vi "PC Streaming Host with slow.vi"() -> ()   [LabVIEW 2012]
uses:
  <vilib>/userdefined/High Color/nirio_resource_hc.ctl
  hv cluster control.ctl
  <vilib>/FPGAPlugInAG/PXI-7951R/niLvFpga_Open_PXI-7951R.vi
  <vilib>/rvi/interface/common/dynamic/niFpgaDynamicAddResources.vi
  <vilib>/Utility/error.llb/Error Cluster From Error Code.vi
  <vilib>/rvi/errors/niLvFpgaAdjustHostInterfaceError.vi
  <vilib>/FPGAPlugInAG/Dynamic/niLvFpga_Close_Dynamic.vi
  <vilib>/rvi/interface/nirviOpenFPGA/nirviOpenFPGA.xnode
  FPGA Bitfiles/TopLevelFPGA3.0.lvbitx
  <vilib>/rvi/interface/nirviReadWriteControl/nirviReadWriteControl.xnode
  <vilib>/rvi/interface/nirviMethod/nirviMethod.xnode
  <vilib>/rvi/interface/nirviCloseFPGA/nirviCloseFPGA.xnode
  <vilib>/ptbypt/NI_PtbyPt.lvlib
  <vilib>/rvi/interface/Simulation/niFpgaSimulationCallBeginRW.vi
  RT_binary.vi
  NiFpgaLv.dll
  <vilib>/FPGAPlugInAG/Dynamic/niLvFpga_ReadFifo_Dynamic.vi
  <vilib>/rvi/errors/niLvFpgaMergeErrorWithErrorCode.vi
  CAENHVs/CAEN/labview/CAENHVWrapper/CAENHVWrapper.lvlib
panel:
  in  "Channel Cluster":T1={"det_type"=["", "", "", "", "", "", "", ""], "Serial numbers"=["", "", "", "", "", "", "", ""], "Sources"=["", "", "", "", "", "", "", ""], "Trigger level"=[4000, 4000, 4000, 4000, 4000, 4000, 4000, 4000], "Data Record On/Off"=[FALSE, FALSE, FALSE, FALSE, FALSE, FALSE, FALSE, FALSE, TRUE, FALSE, FALSE, FALSE, FALSE, FALSE, FALSE, TRUE], "Number of Channels"=8}
  in  "HV Cluster":T2={"HV Power On/Off"=[TRUE, TRUE], "Set Voltage"=["0", "0", "0", "0", "0", "0", "0", "0"], "HV Tolerance (%)"=1.0}
  out "created path":path
  out "File name":string
  out "Total Data Chunks to Write":dbl
  in  "Tab Control":T3(tab)
  in  "Write mode":bool
  out "directory exists - please wait":u8(slide)
  out "directory ok":bool
  in  "Write Enable":bool
  in  "File Path":path=path "D:/Users/reuterc/Desktop"
  out "File Writing Progress (%)":dbl(slide) scale=0.0..100.0
  in  "Slow Control On":bool
  in  "Fast Data On":bool
  in  "Number of Files to Write":u32=1
  in  "IP Address of NIST Time Server":string(combo)
  in  "VISA resource name":refnum<visa-resource-name>="COM3"
  in  "HV Power On/Off":bool[](array[boolean])=[FALSE, FALSE, FALSE, FALSE, FALSE, FALSE, FALSE, FALSE]
  in  "HV Tolerance (%)":dbl=1.0
  out "HV":sgl[](array[numeric])
  in  "IP adress HV2":string="1_0_0"
  in  "IP adress HV1":string="0_0_0"
  out "error HV":errorcluster
  in  "Set Voltage":string[](array[string])=["0", "0", "0", "0", "0", "0", "0", "0"]
  out "handle HV1":i32
  out "handle HV2":i32
  in  "General Cluster":cluster{"Location":i16} {"Location" items=["Purdue", "NIKHEF", "Zurich", "???"]}
  in  "PXI address":T4 caption="RIO Device"
  in  "det_type":string[](array[combo])=["", "", "", "", "", "", "", ""]
  in  "Serial numbers":string[](array[combo])=["", "", "", "", "", "", "", ""]
  in  "Sources":string[](array[combo])=["", "", "", "", "", "", "", ""]
  in  "Trigger level":i16[](array[numeric])=[4000, 4000, 4000, 4000, 4000, 4000, 4000, 4000] caption="Trigger"
  in  "Data Record On/Off":bool[](array[boolean])=[FALSE, FALSE, FALSE, FALSE, FALSE, FALSE, FALSE, FALSE]
  in  "Testpulse Cluster":T5={"Master Pulser On/Off"=FALSE, "Testpulse Turnaround Time (samples)"=14, "Pulse Separation (samples)"=0, "Pulse duration (samples)"=0}
  out "Samples per Data Chunk":u32
  in  "DAQ Info Cluster":T6={"Data Chunks per File"=1000, "Samples per Waveform"=95, "Pretrigger Samples"=15, "circular buffer length (samples)"=1000, "Waveforms per Data Chunk"=5000} {"Waveforms per Data Chunk" format="%.2p"}
  out "Average Throughput":dbl(graph)
  out "Loop Time":u32
  out "Inst. Throughput":dbl format="%#_6p"
  out "Elements in FIFO":u32(graph)
  out "FIFO Overflow":bool
  out "Current Chunk":u32
  out "Current File":i32
  out "Waveform Graph":dynamicdata(graph)
  out "Channel number displayed":i16=-1
  in  "Arduino read rate (Hz)":dbl=1.0
  out "Slow time":u64
  out "data":dbl[](array[numeric])
  in  "XON Character":u8=17 format="%.0x"
  in  "XOFF Character":u8=19 format="%.0x"
  out "Slow Cluster":T7
  out "read buffer":string
  out "Bad sensor?":string
  in  "Max Slow Entries per File":i32=86400
  out "Current Slow File":i32
  out "Current Slow Entry":i32
  out "Sensor out of bounds":bool
  out "Temperature":dbl(graph)
  out "Pressure":dbl(graph)
  out "magnetic field y coordinate":dbl(graph)
  out "total magnetic field":dbl(graph)
  out "magnetic field z coordinate":dbl(graph)
  out "magnetic field x coordinate":dbl(graph)
  out "humidity":dbl(graph)
  out "XML String":string
  out "Slow XML":string
  out "error out":errorcluster
  out "NIST Time":u64
  out "NIST Time Failed to Read":bool
  in  "Minutes to wait":u32=5 min=3
  out "UTC format":bool=TRUE
  out "FPGA Timestamp":u64
  out "Stopped":bool
  in  "stop 2":bool
  in  "stop":bool
  # "Channel 0"
  # "Channel 1"
  # "Channel 2"
  # "Channel 3"
  # "Channel 4"
  # "Channel 5"
  # "Channel 6"
  # "Channel 7"
  # "Write continuously"
  # "Write finite number of files"
  # "Program will stop when number of Files to Write is Complete OR if stop is pressed."
  # "TODO: Make this look like the \"detectors\" tab"
  # "Waveform/Data Chunk information"
  # "To compare directly on a scope: Horizontal scale: 200 ns/div Vertical scale: ~100 mV/div If 15 pretriggers, delay = 700 ns"
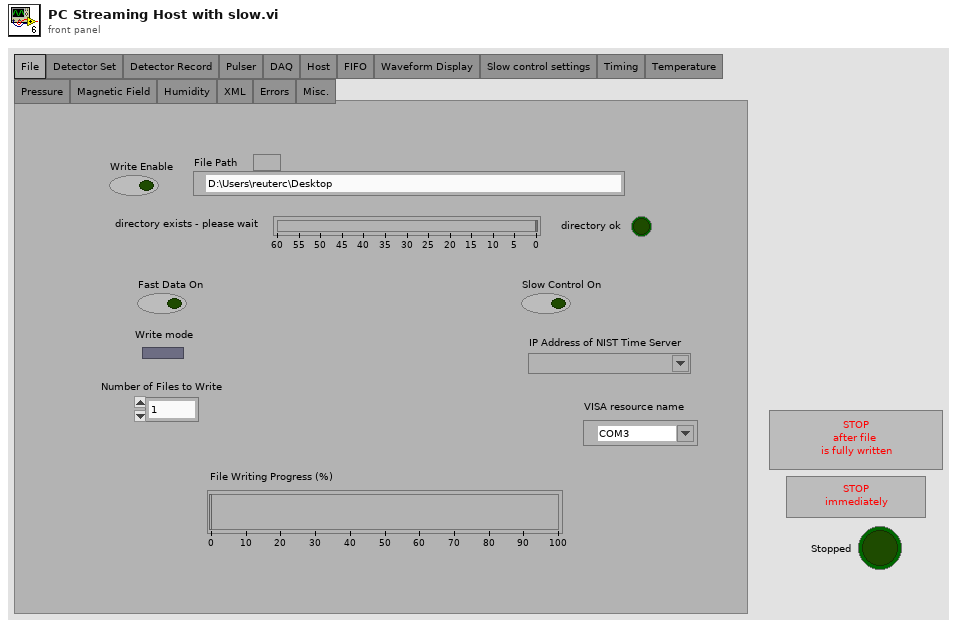
[diagram p1: front panel]
types:
  T1 = cluster{"det_type":string[], "Serial numbers":string[], "Sources":string[], "Trigger level":i16[], "Data Record On/Off":bool[], "Number of Channels":u8}
  T2 = typedef "hv cluster control.ctl" = cluster{"HV Power On/Off":bool[], "Set Voltage":string[], "HV Tolerance (%)":dbl}
  T3 = enum32{"File", "Detector Set", "Detector Record", "Pulser", "DAQ", "Host", "FIFO", "Waveform Display", "Slow control settings", "Timing", "Temperature", "Pressure", "Magnetic Field", "Humidity", "XML", "Errors", "Misc."}
  T4 = typedef "nirio_resource_hc.ctl" = tag
  T5 = cluster{"Master Pulser On/Off":bool, "Testpulse Turnaround Time (samples)":u32, "Pulse Separation (samples)":u32, "Pulse duration (samples)":u32}
  T6 = cluster{"Data Chunks per File":u32, "Samples per Waveform":u32, "Pretrigger Samples":u32, "circular buffer length (samples)":u32, "Waveforms per Data Chunk":u32}
  T7 = cluster{"Arduino Parameters":dbl, "Total Number of Slow Parameters":i32, "UTC format?":bool, "Sensor Upper bounds":i32[], "Sensor Lower bounds":i32[], "Descriptions":string[], "datanames":string[]}
  T8 = enum16{"open", "replace", "create", "open or create", "replace or create", "replace or create with confirmation"}
  T9 = enum16{"big-endian, network order", "native, host order", "little-endian"}
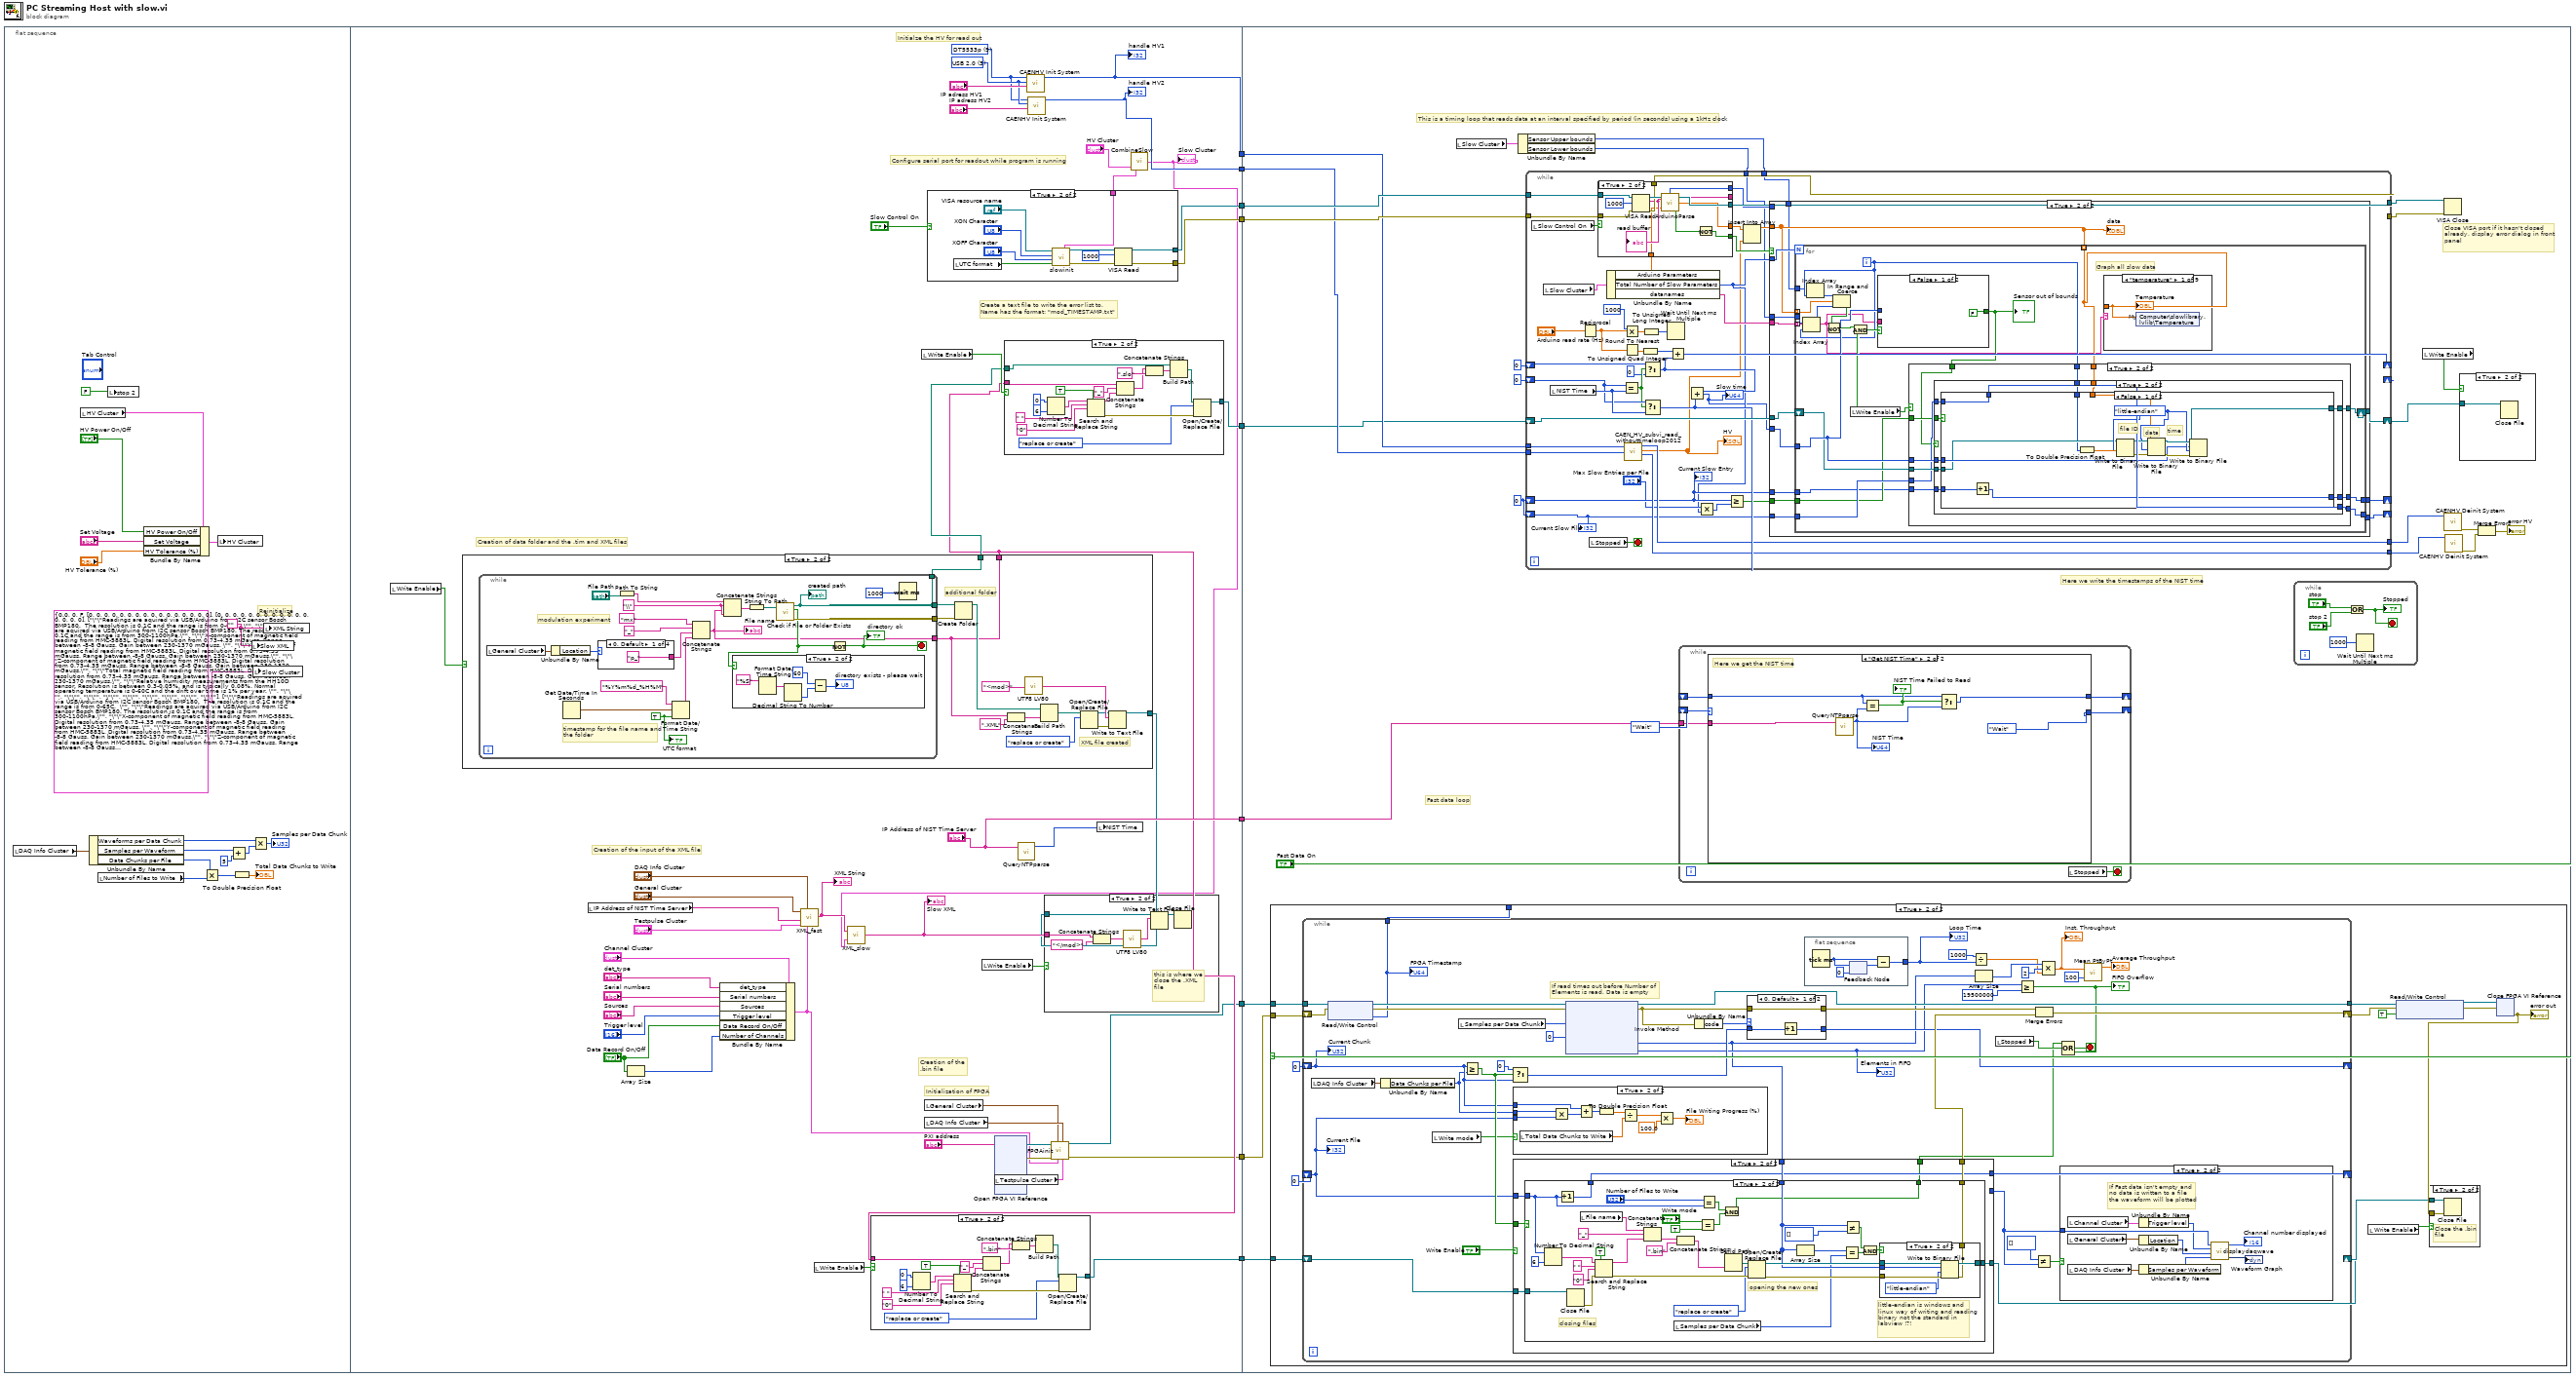
[diagram p0: block diagram]
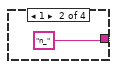
[diagram p7: hidden frame]
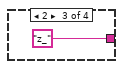
[diagram p8: hidden frame]
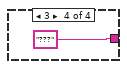
[diagram p9: hidden frame]
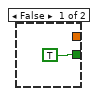
[diagram p11: hidden frame]
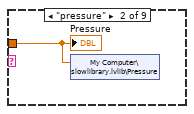
[diagram p13: hidden frame]
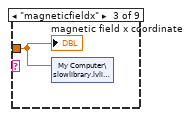
[diagram p14: hidden frame]
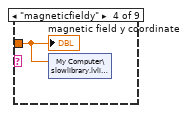
[diagram p15: hidden frame]
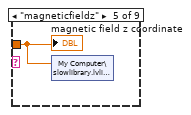
[diagram p16: hidden frame]
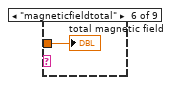
[diagram p17: hidden frame]
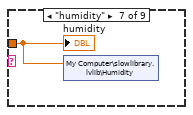
[diagram p18: hidden frame]
diagram:
  n1 = flat-sequence {
    tunnel: ["IP Address of NIST Time Server"] -> w9
    tunnel: [w48] -> w8
    tunnel: [w47] -> w7
    tunnel: [w43] -> w6
    tunnel: [w42] -> w5
    tunnel: [w41] -> w4
    tunnel: [w32] -> w3
    tunnel: [w31] -> w2
    tunnel: [w30] -> w1
    tunnel: w9 -> [w183]
    tunnel: w8 -> [w172]
    tunnel: w7 -> [w171]
    tunnel: w6 -> [w168]
    tunnel: w5 -> [w170]
    tunnel: w4 -> [w169]
    tunnel: w3 -> [w167]
    tunnel: w2 -> [w166]
    tunnel: w1 -> [w165]
    frame #0 {
      w26 = ""
      # "Reinitialize"
      n2 = local read "DAQ Info Cluster"() -> (w19:T6)
      n3 = local read "HV Cluster"() -> (w22:T2)
      n4 = Unbundle By Name(w19) -> ("Waveforms per Data Chunk"=w11:u32, "Samples per Waveform"=w12:u32, "Data Chunks per File"=w13:u32)
      n5 = local read "Number of Files to Write"() -> (w14:u32)
      n6 = local write "stop 2"(FALSE ("stop 2")) -> ()
      n7 = Bundle By Name(cluster=w22, "HV Power On/Off"="HV Power On/Off", "Set Voltage"="Set Voltage", "HV Tolerance (%)"="HV Tolerance (%)") -> (w24:T2)
      n8 = Multiply(x=w13, y=w14) -> (x*y=w18:u32)
      n9 = local write "HV Cluster"(w24) -> ()
      n10 = Add(x=w12, y=u32 5) -> (x+y=w16:u32)
      n11 = To Double Precision Float(number=w18) -> (double precision float=→"Total Data Chunks to Write":dbl)
      n12 = local write "Slow XML"(w26) -> ()
      n13 = Multiply(x=w11, y=w16) -> (x*y=→"Samples per Data Chunk":u32)
      n14 = local write "Slow Cluster"(T7 {"Arduino Parameters"=0.0, "Total Number of Slow Parameters"=0, "UTC format?"=FALSE, "Sensor Upper bounds"=[0, 0, 0, 0, 0, 0, 0, 0, 0, 0, 0, 0, 0, 0, 0, 0], "Sensor Lower bounds"=[0, 0, 0, 0, 0, 0, 0, 0, 0, 0, 0, 0, 0, 0, 0, 0], "Descriptions"=["\"\"Readings are aquired via USB/Arduino from I2C sensor Bosch BMP180.  The resolution is 0.1C and the range is from 0-65C.  \"", "\"\"Readings are aquired via USB/Arduino from I2C sensor Bosch BMP180. The resolution is 0.1C and the range is from 300-1100hPa.\"", "\"\"X-component of magnetic field reading from HMC-5883L. Digital resolution from 0.73-4.35 mGauss. Range between -8-8 Gauss. Gain between 230-1370 mGauss. \"", "\"\"Y-component of magnetic field reading from HMC-5883L. Digital resolution from 0.73-4.35 mGauss. Range between -8-8 Gauss. Gain between 230-1370 mGauss.\"", "\"\"Z-component of magnetic field reading from HMC-5883L. Digital resolution from 0.73-4.35 mGauss. Range between -8-8 Gauss. Gain between 230-1370 mGauss.\"", "\"\"Total magnetic field reading from HMC-5883L. Digital resolution from 0.73-4.35 mGauss. Range between -8-8 Gauss. Gain between 230-1370 mGauss.\"", "\"\"Relative humidity measurements from the HH10D sensor. Resolution is between 0.3-0.05%, and is typically 0.08%. Normal operating temperature is 0-60C and the drift over time is 1% per year. \"", "\"\"", "\"\"", "\"\"", "\"\"", "\"\"", "\"\"", "\"\"", "\"\"", "\"\""], "datanames"=["\"\"Readings are aquired via USB/Arduino from I2C sensor Bosch BMP180.  The resolution is 0.1C and the range is from 0-65C.  \"", "\"\"Readings are aquired via USB/Arduino from I2C sensor Bosch BMP180. The resolution is 0.1C and the range is from 300-1100hPa.\"", "\"\"X-component of magnetic field reading from HMC-5883L. Digital resolution from 0.73-4.35 mGauss. Range between -8-8 Gauss. Gain between 230-1370 mGauss. \"", "\"\"Y-component of magnetic field reading from HMC-5883L. Digital resolution from 0.73-4.35 mGauss. Range between -8-8 Gauss. Gain between 230-1370 mGauss.\"", "\"\"Z-component of magnetic field reading from HMC-5883L. Digital resolution from 0.73-4.35 mGauss. Range between -8-8 Gauss. Gain between 230-1370 mGauss.\"", "\"\"Total magnetic field reading from HMC-5883L. Digital resolution from 0.73-4.35 mGauss. Range between -8-8 Gauss. Gain between 230-1370 mGauss.\"", "\"\"Relative humidity measurements from the HH10D sensor. Resolution is between 0.3-0.05%, and is typically 0.08%. Normal operating temperature is 0-60C and the drift over time is 1% per year. \"", "\"\"", "\"\"", "\"\"", "\"\"", "\"\"", "\"\"", "\"\"", "\"\"", "\"\""]} ("Cluster")) -> ()
      n15 = local write "XML String"(w26) -> ()
    }
    frame #1 {
      w50 = 3 items=["TCP/IP"=0, "HS CAENET"=2, "USB 2.0"=3, "CONET Optical Link"=4, "USB VCP"=5] ("LinkType")
      w49 = u32 9 items=["SY1527", "SY2527", "SY4527", "SY5527", "N568", "V65XX", "N1470", "V8100", "", "DT5533p"] ("system")
      # "Initialization of FPGA"
      # "Creation of the \n.bin file"
      # "Initialze the HV for read out"
      # "Create a text file to write the error list to.  \nName has the format: \"mod_TIMESTAMP.txt\""
      # "Creation of the input of the XML file"
      # "Configure serial port for readout while program is running"
      # "Creation of data folder and the .tim and XML files"
      n16 = local read "Write Enable"() -> (w72:bool)
      n17 = case shown="True" w72 {
        tunnel: [_ w133] -> w44
        tunnel: [_ w125] -> w46
        tunnel: [_ w122] -> w33
        frame False {
        }
        frame True {
          # "XML file created"
          # "additional folder"
          n18 = while {
            tunnel: [w148] -> w134
            tunnel: [w140] -> w135
            tunnel: [w140] -> w133
            tunnel: [w139] -> w122
            stop <- w145 stop-if-true
            w141 = "\\" ("string")
            w151 = TRUE ("UTC format")
            # "modulation experiment"
            # "timestamp for the file name and the folder"
            n19 = local read "General Cluster"() -> (w137:cluster{"Location":i16})
            n20 = Unbundle By Name(w137) -> ("Location"=w136:i16)
            n21 = Get Date/Time In Seconds() -> (seconds since 1Jan1904=w152:timestamp)
            n22 = case shown="0, Default" w136 {
              tunnel: ["p_" ("string") "n_" ("string") "z_" ("string") "???"] -> w138
              frame 0, Default {
              }
              frame 1 {
              }
              frame 2 {
              }
              frame 3 {
              }
            }
            n23 = Path To String(path="File Path") -> (string=w154:string)
            n24 = Format Date/Time String(time format string (%c)="%Y%m%d_%H%M", seconds (now)=w152, UTC format=w151) -> (date/time string=w142:string)
            n25 = Concatenate Strings("mx" ("string"), "_" ("string"), w138, w142) -> (w139:string)
            "File name" <- w139
            n26 = Concatenate Strings(w154, w141, w139, w141) -> (w155:string)
            n27 = String To Path(string=w155) -> (path=w149:path)
            n28 = call <vilib>:"Check if File or Folder Exists.vi"("path"=w149) -> ("error out"=w148:errorcluster, "file or folder exists?"=w147:bool, "dup path"=w140:path)  [unwired: 8 in]
            "created path" <- w140
            n29 = case shown="True" w147 {
              frame False {
              }
              frame True {
                n30 = Format Date/Time String(time format string (%c)="%S") -> (date/time string=w163:string)  [unwired: 2 in]
                n31 = Decimal String To Number(string=w163) -> (number=w161:i32)  [unwired: 2 in, 1 out]
                n32 = Subtract(x=60, y=w161) -> (x-y=→"directory exists - please wait":i32)
              }
            }
            n33 = Not(x=w147) -> (.not. x?=w145:bool)
            "directory ok" <- w145
            n34 = Wait (ms)(milliseconds to wait=1000) -> ()  [unwired: 1 out]
            "UTC format" <- w151
          }
          n35 = Create Folder(path (use dialog)=w135, error in=w134) -> (created path=w123:path)  [unwired: 1 in, 2 out]
          n36 = Concatenate Strings(w122, ".XML" ("substring (\"\")")) -> (w129:string)
          n37 = call "UTF8 LV80.vi"("text"="<mod>") -> ("utf-8 text out"=w132:string)
          n38 = Build Path(base path=w123, name or relative path=w129) -> (appended path=w128:path)
          n39 = Open/Create/Replace File(file path (use dialog)=w128, operation (0:open)=T8."replace or create") -> (refnum out=w131:refnum<file>, error out=w130:errorcluster)  [unwired: 4 in, 1 out]
          n40 = Write to Text File(file (use dialog)=w131, text=w132, error in=w130) -> (refnum out=w125:refnum<file>)  [unwired: 1 in, 2 out]
        }
      }
      n41 = local read "IP Address of NIST Time Server"() -> (w62:string)
      n42 = Array Size(array="Data Record On/Off") -> (size(s)=w60:i32)
      n43 = Bundle By Name(cluster="Channel Cluster", "det_type"="det_type", "Serial numbers"="Serial numbers", "Sources"="Sources", "Trigger level"="Trigger level", "Data Record On/Off"="Data Record On/Off", "Number of Channels"=w60) -> (w29:T1)
      n44 = call "XML_fast.vi"("Channel Cluster"=w29, "DAQ Info Cluster"="DAQ Info Cluster", "Testpulse Cluster"="Testpulse Cluster", "IP Address of NIST Time Server"=w62, "General Cluster"="General Cluster") -> ("XML String"=w65:string)  [unwired: 6 in]
      "XML String" <- w65
      n45 = local read "Write Enable"() -> (w34:bool)
      n46 = case shown="True" w34 {
        tunnel: [_ w81] -> w32
        tunnel: w33 -> [_ w73]
        frame False {
        }
        frame True {
          n47 = Number To Decimal String(number=0, width (-)=i16 6) -> (decimal integer string=w88:string)
          n48 = Search and Replace String(replace all?=TRUE ("replace all? (F)"), input string=w88, search string=" ", replace string="0" ("replace string (\"\")")) -> (result string=w78:string, error out=w83:errorcluster)  [unwired: 4 in, 2 out]
          n49 = Concatenate Strings(w73, "_" ("string"), w78) -> (w76:string)
          n50 = Concatenate Strings(w76, ".bin" ("substring (\"\")")) -> (w80:string)
          n51 = Build Path(name or relative path=w80) -> (appended path=w84:path)  [unwired: 1 in]
          n52 = Open/Create/Replace File(file path (use dialog)=w84, error in=w83, operation (0:open)=T8."replace or create") -> (refnum out=w81:refnum<file>)  [unwired: 3 in, 2 out]
        }
      }
      n53 = local read "Write Enable"() -> (w45:bool)
      n54 = local read "General Cluster"() -> (w37:cluster{"Location":i16})
      n55 = local read "DAQ Info Cluster"() -> (w38:T6)
      n56 = case shown="True" "Slow Control On" {
        tunnel: [_ w121] -> w48
        tunnel: [_ w120] -> w47
        tunnel: [_ w112] -> w71
        frame False {
        }
        frame True {
          n57 = local read "UTC format"() -> (w115:bool)
          n58 = call "slowinit.vi"("UTC format"=w115, "XOFF Character"="XOFF Character", "XON Character"="XON Character", "VISA resource name"="VISA resource name") -> ("error IO"=w113:errorcluster, "VISA resource name out"=w114:refnum<visa-resource-name>, "Slow Cluster"=w112:T7)  [unwired: 5 in]
          n59 = VISA Read(VISA resource name=w114, byte count=u32 1000, error in (no error)=w113) -> (VISA resource name out=w121:refnum<visa-resource-name>, error out=w120:errorcluster)  [unwired: 2 out]
        }
      }
      n60 = local read "Write Enable"() -> (w53:bool)
      n61 = local read "Testpulse Cluster"() -> (w36:T5)
      n62 = xnode "Open FPGA VI Reference"("resource name"="PXI address") -> ("FPGA VI Reference Out"=w40:refnum<k20>, "error out"=w39:errorcluster)  [unwired: 1 in]
      n63 = case shown="True" w45 {
        tunnel: [_ w98] -> w43
        tunnel: w33 -> [_ w90]
        tunnel: w44 -> [_ w89]
        frame False {
        }
        frame True {
          n64 = Number To Decimal String(number=0, width (-)=i16 6) -> (decimal integer string=w105:string)
          n65 = Search and Replace String(replace all?=TRUE ("replace all? (F)"), input string=w105, search string=" ", replace string="0" ("replace string (\"\")")) -> (result string=w95:string, error out=w100:errorcluster)  [unwired: 4 in, 2 out]
          n66 = Concatenate Strings(w90, "_" ("string"), w95) -> (w93:string)
          n67 = Concatenate Strings(w93, ".slo" ("substring (\"\")")) -> (w97:string)
          n68 = Build Path(base path=w89, name or relative path=w97) -> (appended path=w101:path)
          n69 = Open/Create/Replace File(file path (use dialog)=w101, error in=w100, operation (0:open)=T8."replace or create") -> (refnum out=w98:refnum<file>)  [unwired: 3 in, 2 out]
        }
      }
      n70 = call "QueryNTPparse.vi"("IP Address of NIST Server"="IP Address of NIST Time Server") -> ("NTP Time"=w68:u64)  [unwired: 1 in, 2 out]
      n71 = call "CAENHV Init System.vi"("Arg"="IP adress HV1", "LinkType"=w50, "system"=w49) -> ("handle"=w42:i32)  [unwired: 7 in, 1 out]
      "handle HV1" <- w42
      n72 = call "CAENHV Init System.vi"("Arg"="IP adress HV2", "LinkType"=w50, "system"=w49) -> ("handle"=w41:i32)  [unwired: 7 in, 1 out]
      "handle HV2" <- w41
      n73 = call "FPGAinit.vi"("Testpulse Cluster"=w36, "DAQ Info Cluster"=w38, "Channel Cluster"=w29, "General Cluster"=w37, "error in"=w39, "FPGA VI Reference In"=w40) -> ("error out"=w30:errorcluster, "FPGA VI Reference Out"=w31:refnum<k20>)  [unwired: 4 in]
      n74 = local write "NIST Time"(w68) -> ()
      n75 = call "CombineSlow.vi"("HV Cluster"="HV Cluster", "Slow Cluster"=w71) -> ("Slow Cluster 2"=w28:T7)
      "Slow Cluster" <- w28
      n76 = call "XML_slow.vi"("Slow Cluster"=w28, "Input String"=w65) -> ("Output String"=w66:string)
      "Slow XML" <- w66
      n77 = case shown="True" w53 {
        tunnel: w46 -> [_ w111]
        tunnel: w66 -> [_ w106]
        frame False {
        }
        frame True {
          # "this is where we close the .XML file"
          n78 = Concatenate Strings(w106, "</mod>" ("string")) -> (w107:string)
          n79 = call "UTF8 LV80.vi"("text"=w107) -> ("utf-8 text out"=w110:string)
          n80 = Write to Text File(file (use dialog)=w111, text=w110) -> (refnum out=w109:refnum<file>)  [unwired: 2 in, 2 out]
          n81 = Close File(refnum=w109) -> ()  [unwired: 1 in, 2 out]
        }
      }
    }
    frame #2 {
      w173 = 0
      # "Fast data loop"
      # "This is a timing loop that reads data at an interval specified by period (in seconds) using a 1kHz clock"
      # "Close VISA port if it hasn't closed already, display error dialog in front panel"
      # "Here we write the timestamps of the NIST time"
      n82 = case shown="True" "Fast Data On" {
        tunnel: [_ w379] -> _
        tunnel: w167 -> [_ w375]
        tunnel: w166 -> [_ w374]
        tunnel: w165 -> [_ w373]
        frame False {
        }
        frame True {
          n83 = while {
            shift-right: [w416] -> w381
            shift-left: w373 -> [w405]
            shift-right: [w412] -> _
            shift-left: u32 0 -> [w409]
            shift-right: [w397] -> _
            shift-left: 0 ("number") -> [w398]
            shift-right: [w413] -> w383
            shift-left: w375 -> [w414]
            tunnel: [w432] -> w378
            tunnel: [w402] -> w379
            tunnel: w374 -> [w391]
            stop <- w399 stop-if-true
            # "If read times out before Number of Elements is read, Data is empty"
            n84 = local read "DAQ Info Cluster"() -> (w393:T6)
            n85 = xnode "Read/Write Control"("FPGA VI Reference In"=w391, "error in"=w405) -> ("FPGA VI Reference Out"=w404:refnum<k20>, "error out"=w403:errorcluster, "Timestamp"=w402:u64)
            "FPGA Timestamp" <- w402
            n86 = Unbundle By Name(w393) -> ("Data Chunks per File"=w392:u32)
            n87 = local read "Write mode"() -> (w406:bool)
            n88 = local read "Samples per Data Chunk"() -> (w390:u32)
            n89 = Greater Or Equal?(x=w409, y=w392) -> (x >= y?=w418:bool)
            n90 = Select(t=u32 0, s=w418, f=w409) -> (s? t:f=w419:u32)
            n91 = case shown="True" w406 {
              tunnel: w398 -> [_ w451]
              tunnel: w409 -> [_ w449]
              tunnel: w392 -> [_ w442]
              frame False {
              }
              frame True {
                n92 = local read "Total Data Chunks to Write"() -> (w446:dbl)
                n93 = Multiply(x=w442, y=w451) -> (x*y=w450:u32)
                n94 = Add(x=w449, y=w450) -> (x+y=w448:u32)
                n95 = To Double Precision Float(number=w448) -> (double precision float=w447:dbl)
                n96 = Divide(x=w447, y=w446) -> (x/y=w444:dbl)
                n97 = Multiply(x=w444, y=100.0) -> (x*y=→"File Writing Progress (%)":dbl)
              }
            }
            n98 = xnode "Invoke Method"("FPGA VI Reference In"=w404, "error in"=w403, "Number of Elements"=w390, "Timeout (ms)"=0) -> ("FPGA VI Reference Out"=w432:refnum<k20>, "error out"=w429:errorcluster, "Data"=w407:i16[], "Elements Remaining"=w408:u32)
            "Elements in FIFO" <- w408
            n99 = case shown="True" "Write Enable" {
              tunnel: w407 -> [w458 w463]
              tunnel: [w458 _] -> w396
              tunnel: w418 -> [_ w467]
              tunnel: [_ w466] -> w415
              tunnel: [w459 w465] -> w413
              tunnel: w414 -> [w459 w464]
              tunnel: w398 -> [w457 w462]
              tunnel: [w457 w461] -> w397
              tunnel: [FALSE w460] -> w389
              frame False {
              }
              frame True {
                n100 = case shown="True" w467 {
                  tunnel: w463 -> [w471 w495]
                  tunnel: [w470 w497] -> w466
                  tunnel: w464 -> [w475 w510]
                  tunnel: [w474 w503] -> w465
                  tunnel: w462 -> [w469 w484]
                  tunnel: [w469 w490] -> w461
                  tunnel: [FALSE w482] -> w460
                  frame False {
                    # "binary writing will write 0 if there is no data"
                    n101 = Not Equal?(x=w471, y=i16[] []) -> (x != y?=w472:bool)
                    n102 = case shown="True" w472 {
                      tunnel: w475 -> [w476 w481]
                      tunnel: [w476 w480] -> w474
                      tunnel: [_ w479] -> w470
                      tunnel: w471 -> [_ w477]
                      frame False {
                      }
                      frame True {
                        n103 = Write to Binary File(file (use dialog)=w481, data=w477, 9:T9."little-endian" ("byte order (0:big-endian, network order)")) -> (refnum out=w480:refnum<file>, error out=w479:errorcluster)  [unwired: 3 in, 1 out]
                      }
                    }
                  }
                  frame True {
                    # "little-endian is windows and linux way of writing and reading binary not the standard in labview !?!"
                    # "opening the new ones"
                    # "closing files"
                    n104 = Number To Decimal String(number=w484, width (-)=i16 6) -> (decimal integer string=w512:string)
                    n105 = Increment(x=w484) -> (x+1=w490:i32)
                    n106 = Close File(refnum=w510) -> (error out=w509:errorcluster)  [unwired: 1 in, 1 out]
                    n107 = local read "File name"() -> (w491:string)
                    n108 = Search and Replace String(replace all?=TRUE ("replace all? (F)"), input string=w512, search string=" ", replace string="0" ("replace string (\"\")"), error in=w509) -> (result string=w502:string, error out=w508:errorcluster)  [unwired: 3 in, 2 out]
                    n109 = Concatenate Strings(w491, "_" ("string"), w502) -> (w498:string)
                    n110 = local read "Samples per Data Chunk"() -> (w489:u32)
                    n111 = Concatenate Strings(w498, ".bin" ("substring (\"\")")) -> (w500:string)
                    n112 = Equal?(x="Write mode", y=TRUE) -> (x = y?=w488:bool)
                    n113 = Equal?(x="Number of Files to Write", y=w484) -> (x = y?=w487:bool)
                    n114 = And(x=w487, y=w488) -> (x .and. y?=w482:bool)
                    n115 = Build Path(name or relative path=w500) -> (appended path=w507:path)  [unwired: 1 in]
                    n116 = Open/Create/Replace File(file path (use dialog)=w507, error in=w508, operation (0:open)=T8."replace or create") -> (refnum out=w504:refnum<file>, error out=w505:errorcluster)  [unwired: 3 in, 1 out]
                    n117 = Array Size(array=w495) -> (size(s)=w494:i32)
                    n118 = Equal?(x=w494, y=w489) -> (x = y?=w493:bool)
                    n119 = Not Equal?(x=w495, y=i16[] []) -> (x != y?=w496:bool)
                    n120 = And(x=w496, y=w493) -> (x .and. y?=w492:bool)
                    n121 = case shown="True" w492 {
                      tunnel: w505 -> [w517 w524]
                      tunnel: w504 -> [w518 w523]
                      tunnel: [w518 w522] -> w503
                      tunnel: [w517 w521] -> w497
                      tunnel: w495 -> [_ w520]
                      frame False {
                      }
                      frame True {
                        n122 = Write to Binary File(file (use dialog)=w523, data=w520, error in=w524, 9:T9."little-endian" ("byte order (0:big-endian, network order)")) -> (refnum out=w522:refnum<file>, error out=w521:errorcluster)  [unwired: 2 in, 1 out]
                      }
                    }
                  }
                }
              }
            }
            n123 = Unbundle By Name(w429) -> ("code"=w430:i32)
            n124 = case shown="0, Default" w430 {
              tunnel: [w527 errorcluster {"status"=FALSE, "code"=0, "source"=""} ("error constant")] -> w417
              tunnel: w429 -> [w527 _]
              tunnel: w419 -> [w526 w528]
              tunnel: [w525 w528] -> w412
              frame 0, Default {
                n125 = Increment(x=w526) -> (x+1=w525:u32)
              }
              frame -50400 {
                # "Timeout"
              }
            }
            n126 = flat-sequence {
              tunnel: [w455] -> w423
              frame #0 {
                n127 = Tick Count (ms)() -> (millisecond timer value=w454:u32)
                n128 = feedback #1(u32 0 ("millisecond timer value")) -> (w453:u32)
                n129 = feedback-in #1(w454) -> ()
                n130 = Subtract(x=w454, y=w453) -> (x-y=w455:u32)
              }
            }
            n131 = Divide(x=u32 1000, y=w423) -> (x/y=w425:dbl)
            n132 = Array Size(array=w407) -> (size(s)=w428:i32)
            n133 = local read "Stopped"() -> (w401:bool)
            n134 = Greater Or Equal?(x=w408, y=u32 19500000) -> (x >= y?=w400:bool)
            "FIFO Overflow" <- w400
            n135 = Not Equal?(x=i16[] [], y=w396) -> (x != y?=w394:bool)
            n136 = Merge Errors(w417, w415) -> (w416:errorcluster)
            n137 = Compound Arithmetic op=MULTIPLY(w428, 2 ("y"), w425) -> (w422:dbl)
            "Inst. Throughput" <- w422
            n138 = case shown="True" w394 {
              tunnel: w396 -> [_ w441]
              frame False {
              }
              frame True {
                # "If Fast data isn't empty and\nno data is written to a file\nthe waveform will be plotted"
                n139 = local read "Channel Cluster"() -> (w439:T1)
                n140 = local read "General Cluster"() -> (w437:cluster{"Location":i16})
                n141 = local read "DAQ Info Cluster"() -> (w435:T6)
                n142 = Unbundle By Name(w439) -> ("Trigger level"=w438:i16[])
                n143 = Unbundle By Name(w437) -> ("Location"=w436:i16)
                n144 = Unbundle By Name(w435) -> ("Samples per Waveform"=w434:u32)
                n145 = call "displaydaqwave.vi"("Samples per Waveform"=w434, "Location"=w436, "Trigger level"=w438, "Waveform from DAQ"=w441) -> ("Waveform Graph"=→"Waveform Graph":dynamicdata, "Channel number displayed"=→"Channel number displayed":i16)  [unwired: 6 in]
              }
            }
            n146 = Compound Arithmetic op=OR(w389, w401, w400) -> (w399:bool)
            n147 = call <vilib>:"Mean PtByPt.vi"("x"=w422, "sample length"=100) -> ("mean"=→"Average Throughput":dbl)  [unwired: 2 in, 1 out]
            "Loop Time" <- w423
            "Current Chunk" <- w409
            "Current File" <- w398
          }
          n148 = local read "Write Enable"() -> (w385:bool)
          n149 = xnode "Read/Write Control"("FPGA VI Reference In"=w378, "error in"=w381, "Stop FPGA and exit"=TRUE) -> ("FPGA VI Reference Out"=w377:refnum<k20>, "error out"=w376:errorcluster)
          n150 = xnode "Close FPGA VI Reference"("FPGA VI Reference In"=w377, "error in"=w376) -> ("error out"=w386:errorcluster)
          "error out" <- w386
          n151 = case shown="True" w385 {
            tunnel: w386 -> [_ w387]
            tunnel: w383 -> [_ w388]
            frame False {
            }
            frame True {
              # "Close the .bin\nfile"
              n152 = Close File(refnum=w388, error in=w387) -> ()  [unwired: 2 out]
            }
          }
        }
      }
      n153 = local read "Slow Cluster"() -> (w187:T7)
      n154 = Unbundle By Name(w187) -> ("Sensor Upper bounds"=w177:i32[], "Sensor Lower bounds"=w176:i32[])
      n155 = while {
        tunnel: [w236] -> w179
        tunnel: [w235] -> w178
        shift-right: [w228] -> _
        shift-left: u64 0 ("NIST Time") -> [w232]
        shift-right: [w224] -> _
        shift-left: u64 0 -> [w230]
        tunnel: [w216] -> w181
        tunnel: [w215] -> w180
        shift-right: [w208] -> w182
        shift-left: w168 -> [w234]
        shift-right: [w204] -> _
        shift-left: w173 -> [w205]
        shift-right: [w203] -> _
        shift-left: w173 -> [w207]
        tunnel: w177 -> [w196]
        tunnel: w176 -> [w195]
        tunnel: w172 -> [w194]
        tunnel: w171 -> [w193]
        tunnel: w170 -> [w192]
        tunnel: w169 -> [w191]
        stop <- w227 stop-if-true
        n156 = local read "Slow Control On"() -> (w211:bool)
        n157 = local read "Slow Cluster"() -> (w218:T7)
        n158 = local read "NIST Time"() -> (w233:u64)
        n159 = Reciprocal(x="Arduino read rate (Hz)") -> (1/x=w221:dbl)
        n160 = local read "Stopped"() -> (w227:bool)
        n161 = Unbundle By Name(w218) -> ("Arduino Parameters"=w212:dbl, "Total Number of Slow Parameters"=w201:i32, "datanames"=w209:string[])
        n162 = case shown="True" w211 {
          tunnel: [_ w248] -> w236
          tunnel: [_ w247] -> w235
          tunnel: [_ w245] -> w217
          tunnel: [_ w244] -> _
          tunnel: [TRUE w240] -> w210
          tunnel: [_ w242] -> w214
          tunnel: w212 -> [_ w241]
          tunnel: w194 -> [_ w239]
          tunnel: w193 -> [_ w238]
          frame False {
          }
          frame True {
            n163 = VISA Read(VISA resource name=w239, byte count=u32 1000, error in (no error)=w238) -> (VISA resource name out=w248:refnum<visa-resource-name>, read buffer=w246:string, error out=w247:errorcluster)  [unwired: 1 out]
            "read buffer" <- w246
            n164 = call "ArduinoParse.vi"("read buffer"=w246, "Expected Arduino Parameters"=w241) -> ("Number Arduino Parameters"=w245:i32, "Arduino Data Names"=w244:string[], "Arduino Data"=w242:dbl[], "Arduino Read Failed?"=w243:bool)
            n165 = Not(x=w243) -> (.not. x?=w240:bool)
          }
        }
        n166 = Equal?(x=w232, y=w233) -> (x = y?=w231:bool)
        n167 = Multiply(x=u32 1000 ("millisecond multiple"), y=w221) -> (x*y=w223:dbl)
        n168 = Round To Nearest(number=w221) -> (nearest integer value=w220:dbl)
        n169 = call "CAEN_HV_subvi_read_withouttimeloop2012.vi"("handle HV1"=w192, "handle HV2"=w191) -> ("handle HV1 out"=w216:i32, "HV"=w198:sgl[], "handle HV2 out"=w215:i32)  [unwired: 1 in, 1 out]
        "HV" <- w198
        n170 = To Unsigned Quad Integer(1:w220) -> (0:w219:u64)
        n171 = To Unsigned Long Integer(number=w223) -> (unsigned 32bit integer=w222:u32)
        n172 = Select(t=w230, s=w231, f=0) -> (s? t:f=w225:u64)
        n173 = Select(t=w232, s=w231, f=w233) -> (s? t:f=w228:u64)
        n174 = Wait Until Next ms Multiple(millisecond multiple=w222) -> ()  [unwired: 1 out]
        n175 = Add(x=w219, y=w225) -> (x+y=w224:u64)
        n176 = Add(x=w225, y=w228) -> (x+y=w197:u64)
        "Slow time" <- w197
        n177 = Multiply(x="Max Slow Entries per File", y=w201) -> (x*y=w200:i32)
        n178 = Greater Or Equal?(x=w205, y=w200) -> (x >= y?=w206:bool)
        n179 = Insert Into Array(array=w214, new element=w198) -> (w213:dbl[])  [unwired: 1 in]
        n180 = case shown="True" w210 {
          tunnel: w234 -> [w252 w265]
          tunnel: w197 -> [_ w264]
          tunnel: [w252 w261] -> w208
          tunnel: w217 -> [_ _]
          tunnel: w213 -> [_ w255]
          tunnel: w209 -> [_ w263]
          tunnel: w201 -> [_ w262]
          tunnel: w207 -> [w250 w260]
          tunnel: w206 -> [_ w259]
          tunnel: w205 -> [w251 w258]
          tunnel: [w251 w257] -> w204
          tunnel: [w250 w256] -> w203
          tunnel: w196 -> [_ w254]
          tunnel: w195 -> [_ w253]
          frame False {
          }
          frame True {
            n181 = for {
              N: w262 -> [_]
              tunnel: w264 -> [w282]
              tunnel: w255 -> [w285] mode=indexing
              tunnel: w263 -> [w270] mode=indexing
              tunnel: w255 -> [w271] mode=indexing
              tunnel: w260 -> [w279]
              tunnel: w259 -> [w277]
              tunnel: w258 -> [w276]
              tunnel: [w275] -> w257
              tunnel: [w274] -> w256
              shift-right: [w280] -> w261
              shift-left: w265 -> [w281]
              tunnel: w254 -> [w269]
              tunnel: w253 -> [w268]
              i -> [w278]
              # "Graph all slow data"
              n182 = Index Array(array=w268, index=w278) -> (element=w267:i32)
              n183 = Index Array(array=w269, index=w278) -> (element=w266:i32)
              n184 = In Range and Coerce(upper limit=w266, x=w285, lower limit=w267) -> (In Range?=w273:bool)  [unwired: 1 out]
              n185 = Not(x=w273) -> (.not. x?=w286:bool)
              n186 = local read "Write Enable"() -> (w283:bool)
              n187 = And(x=w286, y=w283) -> (x .and. y?=w284:bool)
              n188 = case shown="False" w284 {
                tunnel: w270 -> [_ w366]
                tunnel: w282 -> [_ _]
                tunnel: [FALSE ("Sensor out of bounds") TRUE ("Sensor out of bounds")] -> w272
                frame False {
                }
                frame True {
                  "Bad sensor?" <- w366
                }
              }
              "Sensor out of bounds" <- w272
              n189 = case shown="True" w283 {
                tunnel: [w294 w307] -> w274
                tunnel: w271 -> [_ w306]
                tunnel: w282 -> [_ w305]
                tunnel: w281 -> [w296 w304]
                tunnel: [w296 w303] -> w280
                tunnel: w279 -> [w294 w302]
                tunnel: w278 -> [_ w301]
                tunnel: w277 -> [_ w300]
                tunnel: w276 -> [w295 w299]
                tunnel: [w295 w298] -> w275
                tunnel: w272 -> [_ w297]
                frame False {
                }
                frame True {
                  n190 = case shown="True" w297 {
                    tunnel: [w309 w320] -> w307
                    tunnel: w306 -> [_ w319]
                    tunnel: w305 -> [_ w318]
                    tunnel: w304 -> [w308 w317]
                    tunnel: [w308 w316] -> w303
                    tunnel: w302 -> [w309 w315]
                    tunnel: w301 -> [_ w314]
                    tunnel: w300 -> [_ w313]
                    tunnel: w299 -> [w310 w312]
                    tunnel: [w310 w311] -> w298
                    frame False {
                    }
                    frame True {
                      n191 = case shown="False" w313 {
                        tunnel: [w324 w336] -> w320
                        tunnel: w319 -> [w328 w344]
                        tunnel: w318 -> [w327 w343]
                        tunnel: w317 -> [w325 w342]
                        tunnel: [w326 w340] -> w316
                        tunnel: w315 -> [w324 w339]
                        tunnel: w314 -> [w323 w338]
                        tunnel: w312 -> [w322 _]
                        tunnel: [w321 0] -> w311
                        frame False {
                          w329 = T9."little-endian" ("byte order (0:big-endian, network order)")
                          # "time"
                          # "data"
                          # "file ID"
                          n192 = Increment(x=w322) -> (x+1=w321:i32)
                          n193 = To Double Precision Float(number=w323) -> (double precision float=w330:dbl)
                          n194 = Write to Binary File(file (use dialog)=w325, data=w330, 9:w329) -> (refnum out=w333:refnum<file>, error out=w334:errorcluster)  [unwired: 3 in, 1 out]
                          n195 = Write to Binary File(file (use dialog)=w333, data=w328, error in=w334, 9:w329) -> (refnum out=w332:refnum<file>, error out=w331:errorcluster)  [unwired: 2 in, 1 out]
                          n196 = Write to Binary File(file (use dialog)=w332, data=w327, error in=w331, 9:w329) -> (refnum out=w326:refnum<file>)  [unwired: 2 in, 2 out]
                        }
                        frame True {
                          w345 = T9."little-endian" ("byte order (0:big-endian, network order)")
                          w335 = TRUE ("replace all? (F)")
                          # "time"
                          # "data"
                          # "file ID"
                          # "opening the new ones"
                          # "closing files"
                          n197 = local read "File name"() -> (w351:string)
                          n198 = Increment(x=w339) -> (x+1=w336:i32)
                          n199 = Number To Decimal String(number=w336, width (-)=i16 6) -> (decimal integer string=w361:string)
                          n200 = Close File(refnum=w342) -> (error out=w359:errorcluster)  [unwired: 1 in, 1 out]
                          n201 = Search and Replace String(replace all?=w335, case sensitive?=w335, input string=w361, search string=" ", replace string="0" ("replace string (\"\")"), error in=w359) -> (result string=w355:string, error out=w358:errorcluster)  [unwired: 2 in, 2 out]
                          n202 = Concatenate Strings(w351, "_" ("string"), w355) -> (w352:string)
                          n203 = Concatenate Strings(w352, ".slo" ("substring (\"\")")) -> (w353:string)
                          n204 = Build Path(name or relative path=w353) -> (appended path=w357:path)  [unwired: 1 in]
                          n205 = Open/Create/Replace File(file path (use dialog)=w357, error in=w358, operation (0:open)=T8."replace or create") -> (refnum out=w341:refnum<file>)  [unwired: 3 in, 2 out]
                          n206 = To Double Precision Float(number=w338) -> (double precision float=w346:dbl)
                          n207 = Write to Binary File(file (use dialog)=w341, data=w346, 9:w345) -> (refnum out=w349:refnum<file>, error out=w350:errorcluster)  [unwired: 3 in, 1 out]
                          n208 = Write to Binary File(file (use dialog)=w349, data=w344, error in=w350, 9:w345) -> (refnum out=w348:refnum<file>, error out=w347:errorcluster)  [unwired: 2 in, 1 out]
                          n209 = Write to Binary File(file (use dialog)=w348, data=w343, error in=w347, 9:w345) -> (refnum out=w340:refnum<file>)  [unwired: 2 in, 2 out]
                        }
                      }
                    }
                  }
                }
              }
              n210 = case shown="\"temperature\"" w270 {
                tunnel: w271 -> [w287 w288 w289 w290 w291 w292 w293 _ _]
                frame "temperature" {
                  n211 = shared-variable "My Computer\\slowlibrary.lvlib\\Temperature"(w287) -> ()  [unwired: 1 in, 1 out]
                  "Temperature" <- w287
                }
                frame "pressure" {
                  n212 = shared-variable "My Computer\\slowlibrary.lvlib\\Pressure"(w288) -> ()  [unwired: 1 in, 1 out]
                  "Pressure" <- w288
                }
                frame "magneticfieldx" {
                  n213 = shared-variable "My Computer\\slowlibrary.lvlib\\B_x"(w289) -> ()  [unwired: 1 in, 1 out]
                  "magnetic field x coordinate" <- w289
                }
                frame "magneticfieldy" {
                  n214 = shared-variable "My Computer\\slowlibrary.lvlib\\B_y"(w290) -> ()  [unwired: 1 in, 1 out]
                  "magnetic field y coordinate" <- w290
                }
                frame "magneticfieldz" {
                  n215 = shared-variable "My Computer\\slowlibrary.lvlib\\B_z"(w291) -> ()  [unwired: 1 in, 1 out]
                  "magnetic field z coordinate" <- w291
                }
                frame "magneticfieldtotal" {
                  "total magnetic field" <- w292
                }
                frame "humidity" {
                  n216 = shared-variable "My Computer\\slowlibrary.lvlib\\Humidity"(w293) -> ()  [unwired: 1 in, 1 out]
                  "humidity" <- w293
                }
                frame "seconds" {
                }
                frame "", Default {
                }
              }
            }
            "data" <- w255
          }
        }
        "Current Slow Entry" <- w205
        "Current Slow File" <- w207
      }
      n217 = while {
        shift-right: [w534] -> _
        shift-left: enum16{"Wait", "Get NIST Time", "Write"}."Wait" -> [w535]
        shift-right: [w533] -> _
        shift-left: _ -> [w532]
        tunnel: w183 -> [w531]
        stop <- w530 stop-if-true
        n218 = case shown="\"Get NIST Time\"" w535 {
          tunnel: [w538 enum16{"Wait", "Get NIST Time", "Write"}."Wait"] -> w534
          tunnel: [w537 w553] -> w533
          tunnel: w532 -> [w537 w550]
          tunnel: w531 -> [_ w549]
          frame "Wait", Default {
            # "First we wait 'minutes to wait' and proceed with Getting the NIST time\nthis is necessary to see a  drift, if it is there, between the PFGA and NIST time"
            n219 = while {
              tunnel: [enum16{"Wait", "Get NIST Time", "Write"}."Get NIST Time"] -> w538
              tunnel: "Minutes to wait" -> [w540]
              i -> [w543]
              stop <- w544 stop-if-true
              n220 = Multiply(x=60, y=w540) -> (x*y=w539:u32)
              n221 = local read "Stopped"() -> (w542:bool)
              n222 = Wait Until Next ms Multiple(millisecond multiple=u32 1000 ("y")) -> ()  [unwired: 1 out]
              n223 = Greater Or Equal?(x=w543, y=w539) -> (x >= y?=w545:bool)
              n224 = Or(x=w545, y=w542) -> (x .or. y?=w544:bool)
            }
          }
          frame "Get NIST Time" {
            # "Here we get the NIST time"
            n225 = call "QueryNTPparse.vi"("IP Address of NIST Server"=w549) -> ("NTP Time"=w552:u64)  [unwired: 1 in, 2 out]
            "NIST Time" <- w552
            n226 = Equal?(x=w550, y=w552) -> (x = y?=w551:bool)
            "NIST Time Failed to Read" <- w551
            n227 = Select(t=w550, s=w551, f=w552) -> (s? t:f=w553:u64)
          }
        }
        n228 = local read "Stopped"() -> (w530:bool)
      }
      n229 = while {
        stop <- w369 stop-if-true
        n230 = Or(x="stop", y="stop 2") -> (x .or. y?=w369:bool)
        "Stopped" <- w369
        n231 = Wait Until Next ms Multiple(millisecond multiple=u32 1000 ("y")) -> ()  [unwired: 1 out]
      }
      n232 = local read "Write Enable"() -> (w188:bool)
      n233 = VISA Close(VISA resource name=w179, error in (no error)=w178) -> ()  [unwired: 1 out]
      n234 = call "CAENHV Deinit System.vi"("handle"=w181) -> ("error out"=w186:errorcluster)  [unwired: 10 in]
      n235 = call "CAENHV Deinit System.vi"("handle"=w180) -> ("error out"=w185:errorcluster)  [unwired: 10 in]
      n236 = case shown="True" w188 {
        tunnel: w182 -> [_ w368]
        frame False {
        }
        frame True {
          n237 = Close File(refnum=w368) -> ()  [unwired: 1 in, 2 out]
        }
      }
      n238 = Merge Errors(w186, w185) -> (→"error HV":errorcluster)
    }
  }
